vi "Read vRegistry.vi"(8 "error in (no error)":errorcluster, 11 "CloneRegistration in":refnum<class "CloneRegistration.lvclass">) -> (0 "error out":errorcluster, 2 "vRegistry":variant, 3 "CloneRegistration out":refnum<class "CloneRegistration.lvclass">)   [LabVIEW 2018, in "ModuleAdmin.lvlib" / "CloneRegistration.lvclass"]
uses:
  CloneRegistration.lvclass
  CloneRegistration.lvclass/CloneRegistration.ctl
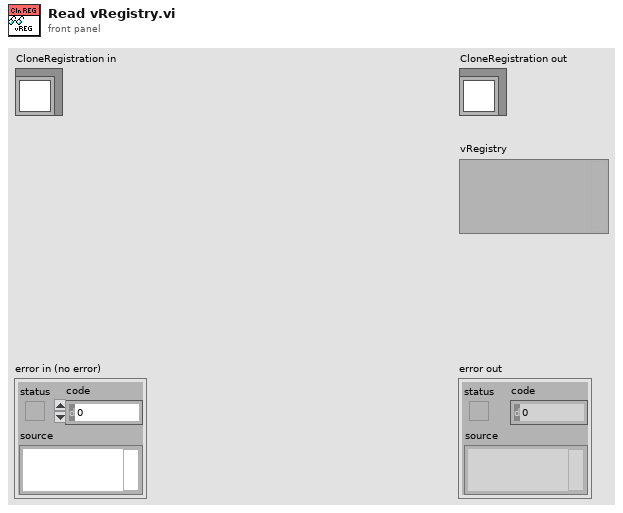
[diagram p1: front panel]
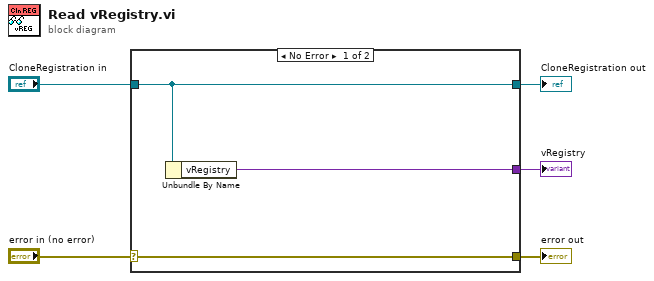
[diagram p0: block diagram]
diagram:
  n1 = case shown="No Error" "error in (no error)" {
    selector: "error in (no error)" -> [w8 w9]
    tunnel: [w8 w9] -> w4
    tunnel: [w7 w10] -> w2
    tunnel: "CloneRegistration in" -> [w7 w10]
    tunnel: [w6 _] -> w1
    frame No Error {
      n2 = Unbundle By Name(w7) -> ("vRegistry"=w6:variant)
    }
    frame Error {
    }
  }
  "error out" <- w4
  "CloneRegistration out" <- w2
  "vRegistry" <- w1
